vi "XLP80_EA_WriteOutputs_Stack.vi"(8 "err in":errorcluster, 11 "Device information":string[](array[string])=["ASRL1::INSTR", "EL 3160-60 A", "000", "///", "1", "160", "60", "400", "10", "400"]) -> (0 "err out":errorcluster, 3 "Device information IN":string[](array[string])=["ASRL1::INSTR", "EL 3160-60 A", "000", "///", "1", "160", "60", "400", "10", "400"])   [LabVIEW 2021]
uses:
  XLP80_EA_Globals.vi
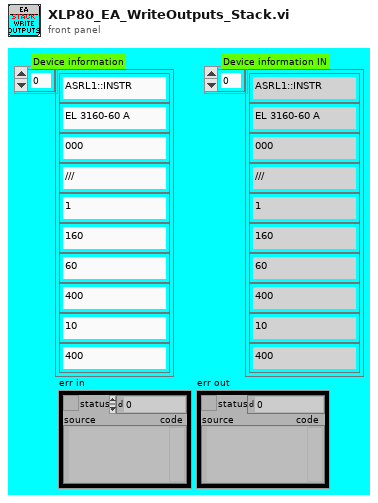
[diagram p1: front panel]
types:
  T1 = typedef "XLP80_EA_TDefsCluster_EA Setpoint.ctl" = cluster{"Load":bool, "Set Current":sgl, "Set Voltage":sgl}
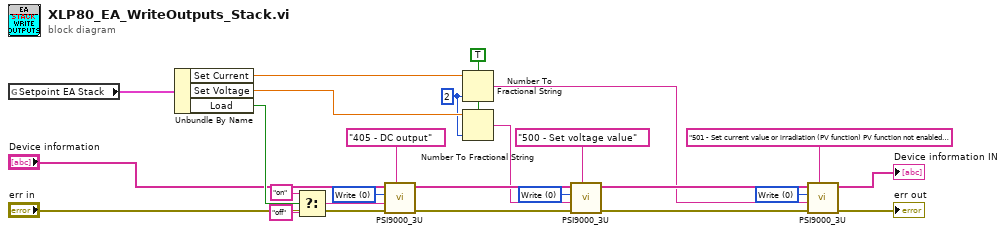
[diagram p0: block diagram]
diagram:
  w7 = u8 0 items=["Write", "Read"] ("Access")
  w8 = u8 0 items=["Write", "Read"] ("Access")
  w6 = TRUE ("use system decimal point (T)")
  w1 = i16 2 ("precision (6)")
  w20 = u8 0 items=["Write", "Read"] ("Access")
  n1 = global read "XLP80_EA_Globals.vi" "Setpoint EA Stack"() -> (w25:T1)
  n2 = Unbundle By Name(w25) -> ("Set Current"=w5:sgl, "Set Voltage"=w21:sgl, "Load"=w24:bool)
  n3 = Select(t="on" ("Value"), s=w24, f="off") -> (s? t:f=w19:string)
  n4 = call <instrlib>:"PSI9000_3U.vi"("Command list"="405 - DC output", "Error in"="err in", "Value"=w19, "Access"=w20, "Device information in"="Device information") -> ("Error out"=w13:errorcluster, "Device information out"=w14:string[])  [unwired: 1 in, 2 out]
  n5 = Number To Fractional String(use system decimal point (T)=w6, number=w5, precision (6)=w1) -> (F-format string=w9:string)  [unwired: 1 in]
  n6 = Number To Fractional String(use system decimal point (T)=w6, number=w21, precision (6)=w1) -> (F-format string=w10:string)  [unwired: 1 in]
  n7 = call <instrlib>:"PSI9000_3U.vi"("Command list"="500 - Set voltage value", "Error in"=w13, "Value"=w10, "Access"=w8, "Device information in"=w14) -> ("Error out"=w12:errorcluster, "Device information out"=w11:string[])  [unwired: 1 in, 2 out]
  n8 = call <instrlib>:"PSI9000_3U.vi"("Command list"="501 - Set current value or irradiation (PV function) PV function not enabled for PSB/PSBEE PSB/PSBE 9000: source mode", "Error in"=w12, "Value"=w9, "Access"=w7, "Device information in"=w11) -> ("Error out"=→"err out":errorcluster, "Device information out"=→"Device information IN":string[])  [unwired: 1 in, 2 out]
